vi "Database Configuration.vi"() -> ()   [LabVIEW 2023, in "GUI.lvlib" / "Diagnostic.lvlib"]
uses:
  Diagnostic.lvlib
  HardwareAbstractionLayer_LVOOP/Database/SQL Public VI/Control/DB Options.ctl
  <vilib>/Utility/file.llb/Write Delimited Spreadsheet (string).vi
  <vilib>/Utility/file.llb/Read Delimited Spreadsheet (string).vi
  HardwareAbstractionLayer_LVOOP/Database/Database.lvclass
panel:
  out "PhysicalChannel":string
  in  "Search":bool
  in  "Update":bool
  in  "Tab Control":enum32{"DAQ", "Database"}(tab)
  in  "DAQ":i32(listbox)
  in  "Signal Name":string(combo)
  in  "Enabled":bool
  in  "Channel Type":string(combo)
  in  "DUT ID":string(combo)
  in  "List Table Name":string(combo)
  in  "List Schema":string(combo)
  in  "Selection":string(combo)
  in  "Export":bool
  in  "Import":bool
  in  "Database":i32(listbox)
  in  "Exit":bool
  out "error out":errorcluster
  in  "error in":errorcluster
  # "Database Configuration"
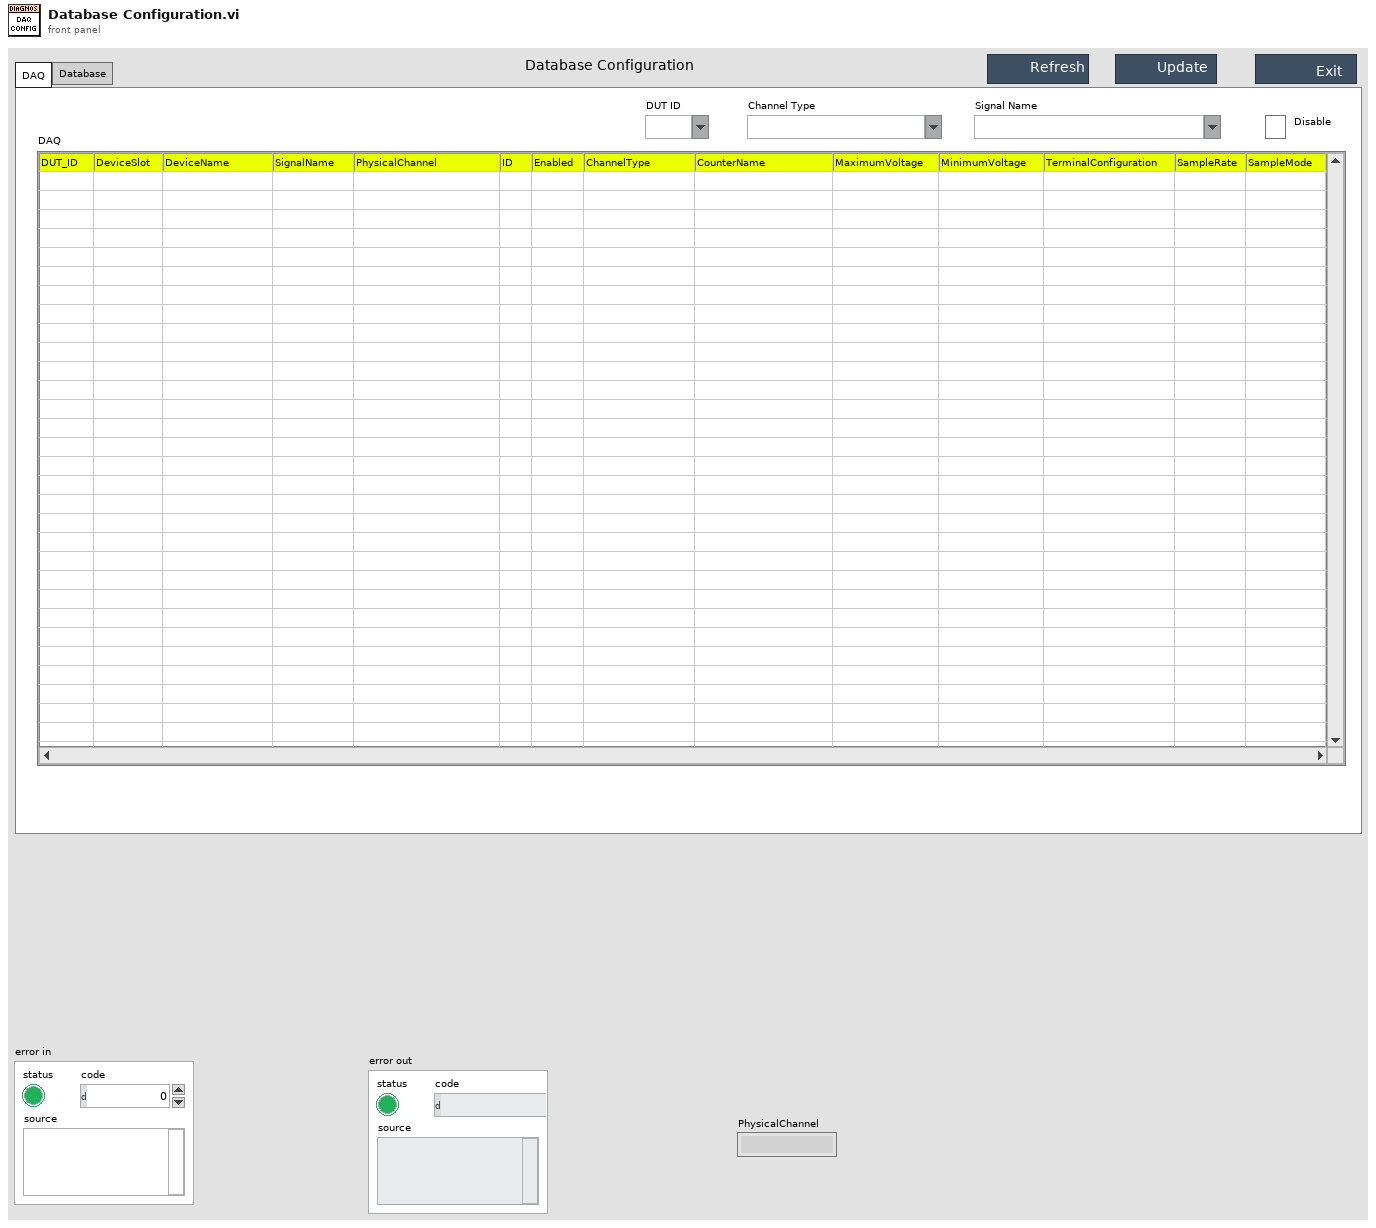
[diagram p1: front panel]
types:
  T1 = typedef "HardwareAbstractionLayer_LVOOP.lvlib/Database.lvclass/DB Options.ctl" = enum16{"Init", "Select Data", "Insert Data", "Update Data", "Delete Data", "Execute Query", "Create Schema", "Create Table", "List Tables", "List Columns", "Close"}
  T2 = cluster{"table":string, "columns":string[], "Data":string[][], "Schema Name":string}
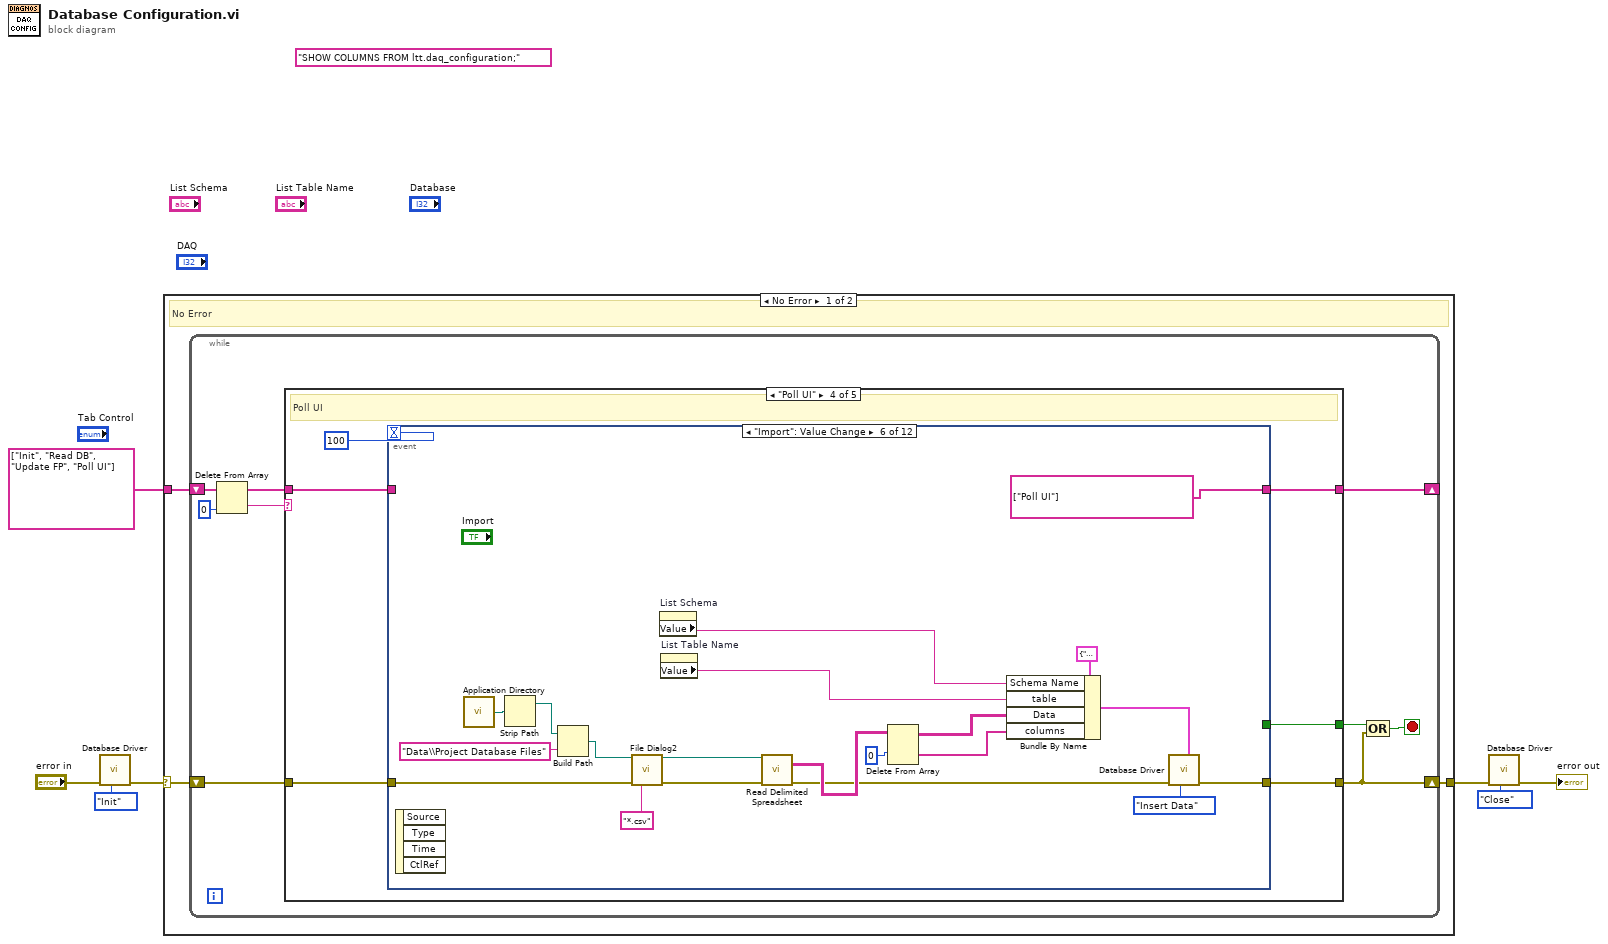
[diagram p0: block diagram]
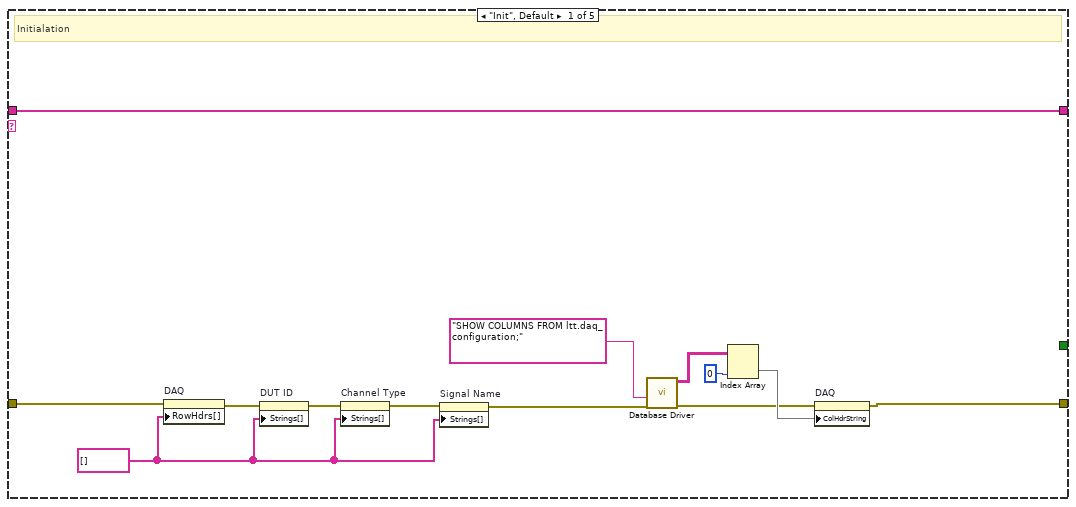
[diagram p2: hidden frame]
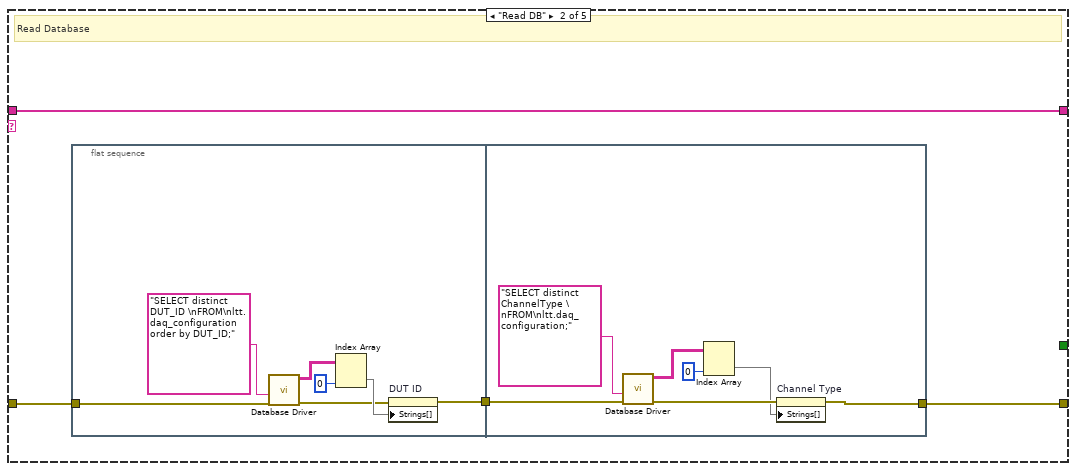
[diagram p3: hidden frame]
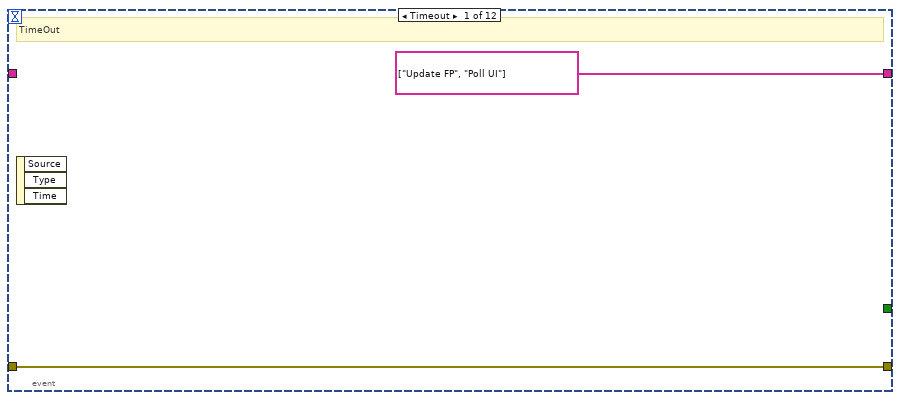
[diagram p5: hidden frame]
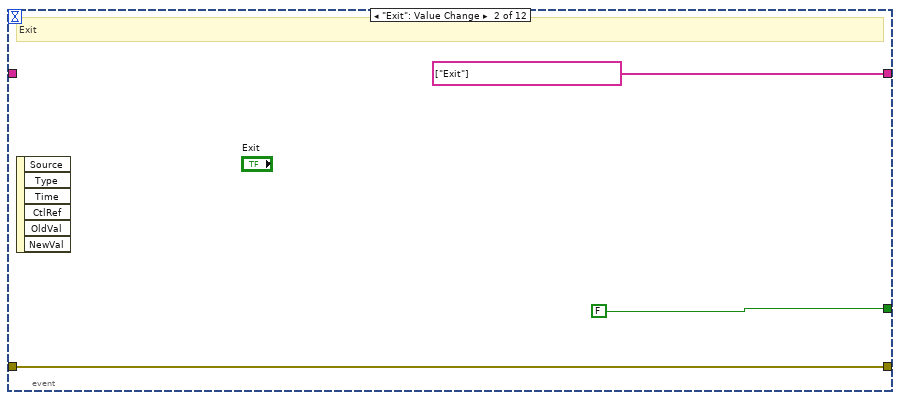
[diagram p6: hidden frame]
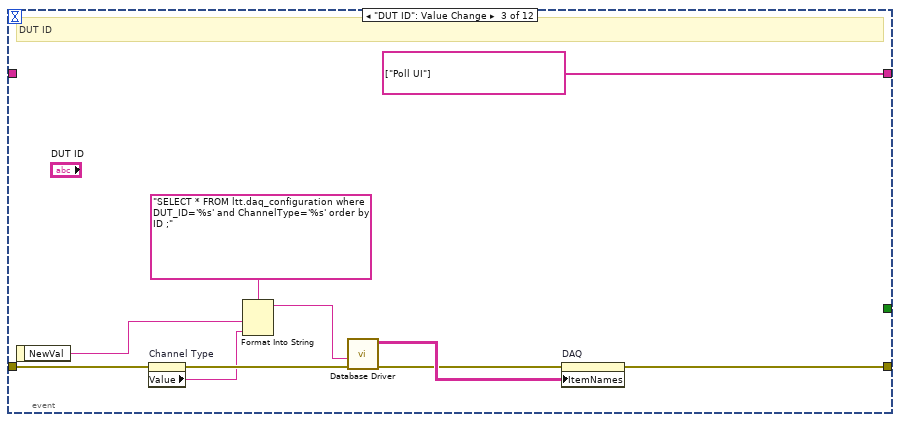
[diagram p7: hidden frame]
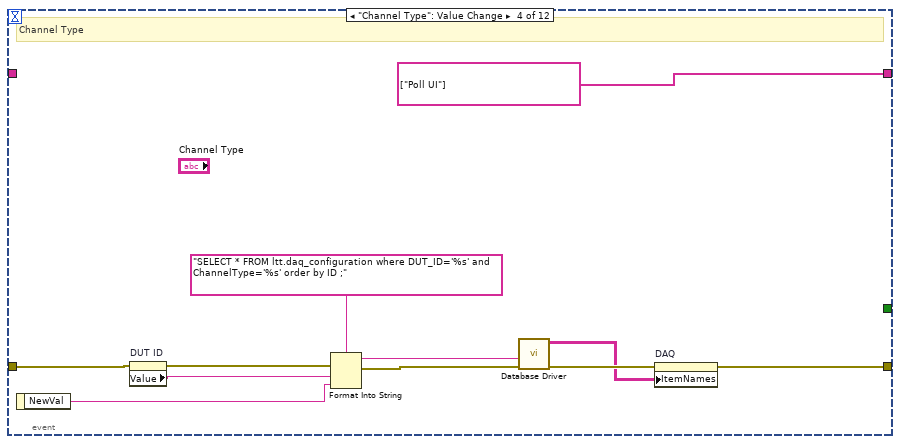
[diagram p8: hidden frame]
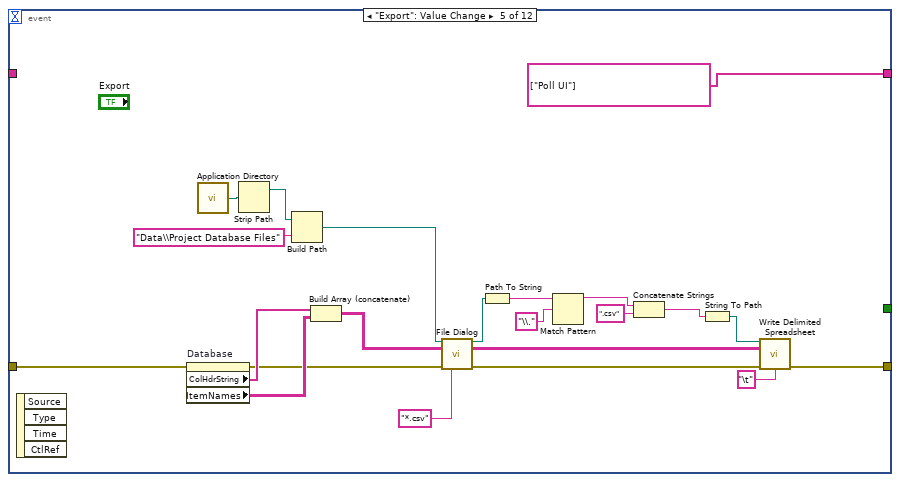
[diagram p9: hidden frame]
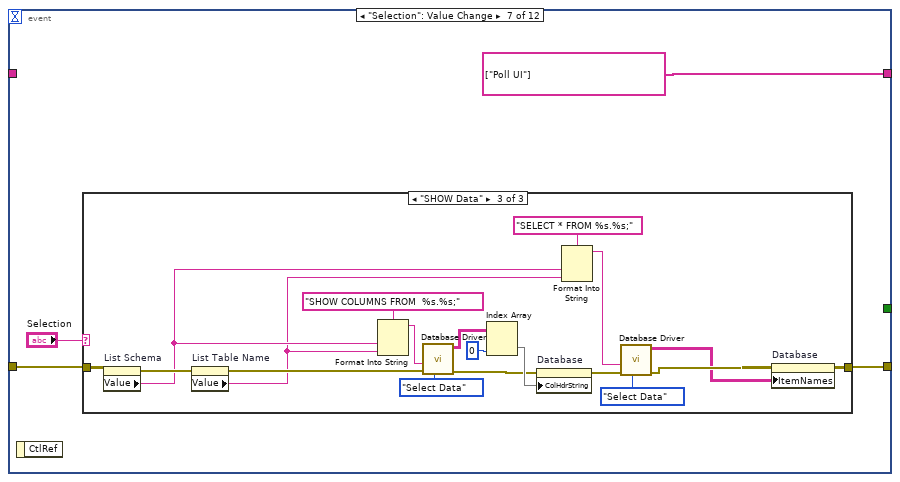
[diagram p10: hidden frame]
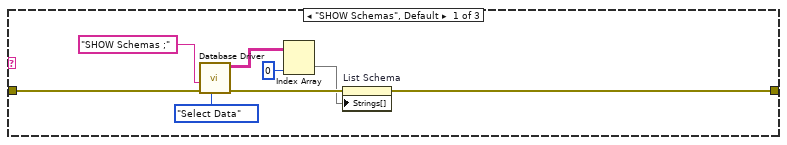
[diagram p11: hidden frame]
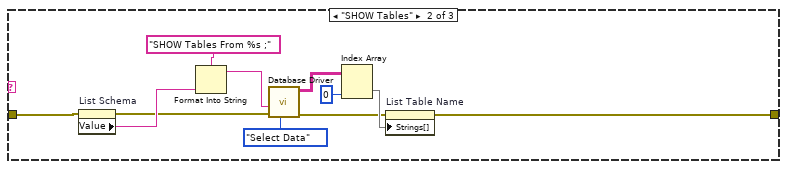
[diagram p12: hidden frame]
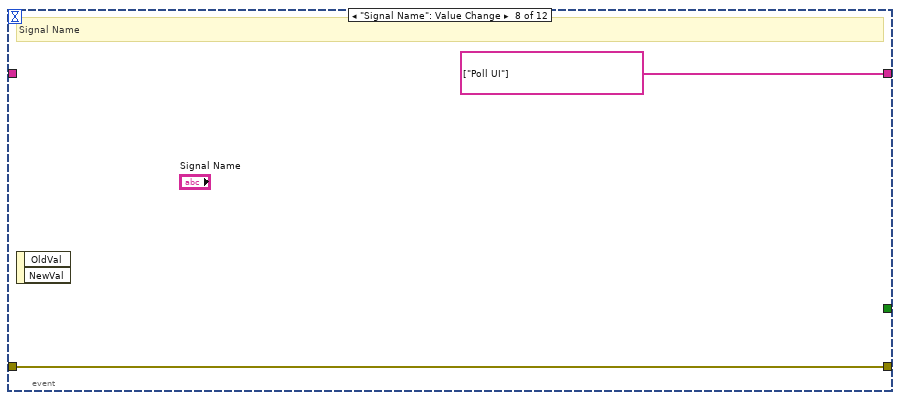
[diagram p13: hidden frame]
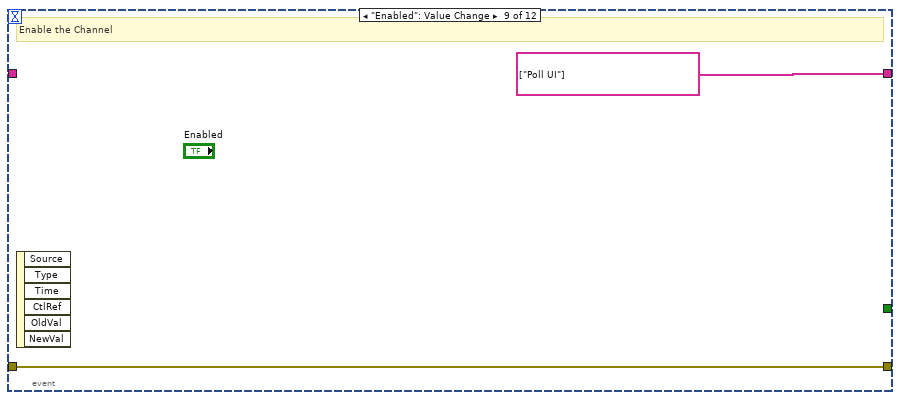
[diagram p14: hidden frame]
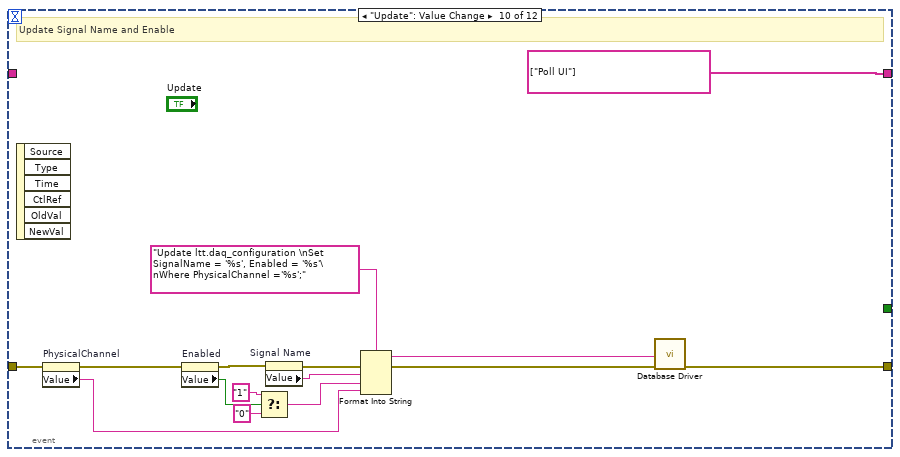
[diagram p15: hidden frame]
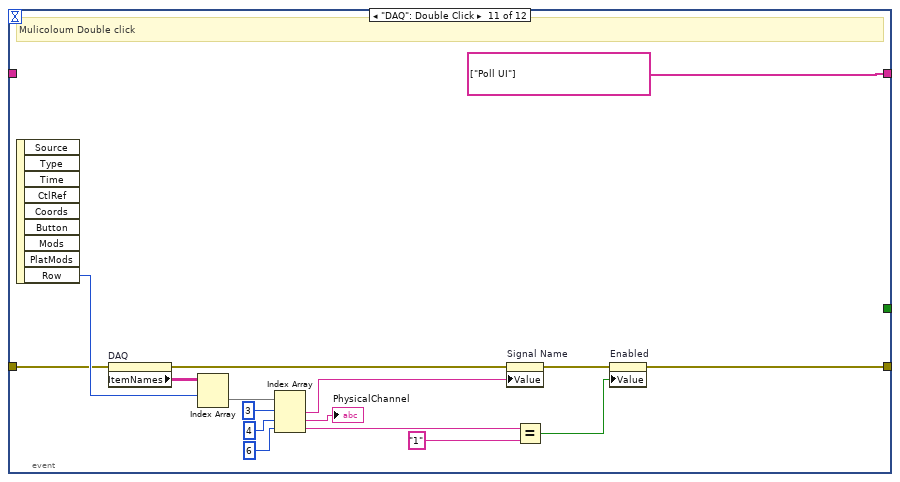
[diagram p16: hidden frame]
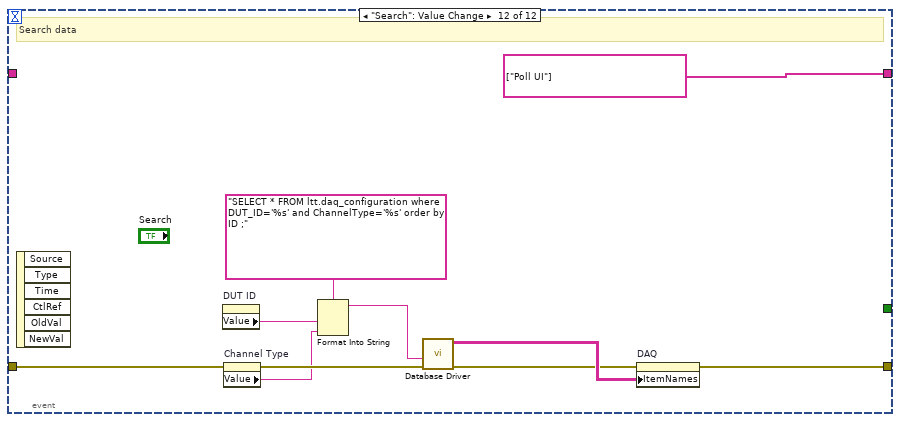
[diagram p17: hidden frame]
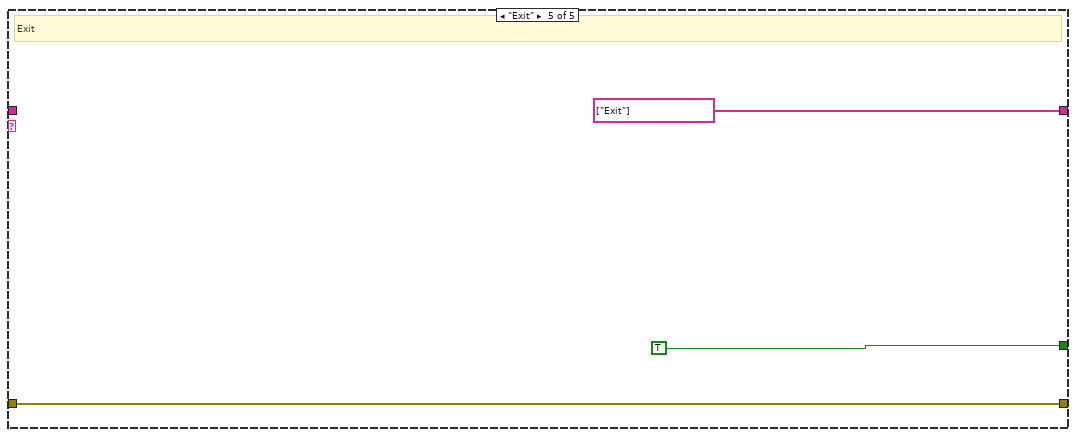
[diagram p18: hidden frame]
diagram:
  (unwired) "SHOW COLUMNS FROM ltt.daq_configuration;" ("SQL query")
  n1 = call "Database Driver.vi"("Options"=DB_Options."Init", "error in"="error in") -> ("error out"=w3:errorcluster)  [unwired: 6 in, 3 out]
  n2 = case shown="No Error" w3 {
    selector: w3 -> [w10 w216]
    tunnel: [w9 w216] -> w2
    tunnel: string[] ["Init", "Read DB", "Update FP", "Poll UI"] -> [w8 _]
    frame No Error {
      # "No Error"
      n3 = while {
        shift-right: [w11] -> w9
        shift-left: w10 -> [w19]
        shift-right: [w15] -> _
        shift-left: w8 -> [w18]
        stop <- w12 stop-if-true
        n4 = Delete From Array(array=w18, index=0) -> (deleted portion=w17:string, array with subset deleted=w16:string[])  [unwired: 1 in]
        n5 = case shown="\"Poll UI\"" w17 {
          tunnel: w19 -> [w31 w35 w51 w58 w214]
          tunnel: [w20 w34 w51 w57 w214] -> w11
          tunnel: w16 -> [w32 w36 w52 w54 _]
          tunnel: [w32 w36 w52 w53 string[] ["Exit"]] -> w15
          tunnel: [_ _ _ w55 TRUE] -> w14
          frame "Init", Default {
            w27 = string[] [] ("Row Header Strings[]")
            # "Initialation"
            n6 = property on="DAQ" class="MCListbox (strict)"(error in=w31, "RowHdrs[]"=w27) -> (error out=w30:errorcluster)  [unwired: 1 in, 1 out]
            n7 = property on="DUT ID" class="CmbBox"(error in=w30, "Strings[]"=w27) -> (error out=w29:errorcluster)  [unwired: 1 in, 1 out]
            n8 = property on="Channel Type" class="CmbBox"(error in=w29, "Strings[]"=w27) -> (error out=w28:errorcluster)  [unwired: 1 in, 1 out]
            n9 = property on="Signal Name" class="CmbBox"(error in=w28, "Strings[]"=w27) -> (error out=w26:errorcluster)  [unwired: 1 in, 1 out]
            n10 = call "Database Driver.vi"("error in"=w26, "SQL query"="SHOW COLUMNS FROM ltt.daq_configuration;") -> ("error out"=w21:errorcluster, "data"=w24:string[][])  [unwired: 6 in, 2 out]
            n11 = Index Array(array=w24, index (col)=0 ("disabled index (col)")) -> (element=w22:string[])  [unwired: 1 in]
            n12 = property on="DAQ" class="MCListbox (strict)"(error in=w21, "ColHdrString"=w22) -> (error out=w20:errorcluster)  [unwired: 1 in, 1 out]
          }
          frame "Read DB" {
            # "Read Database"
            n13 = flat-sequence {
              tunnel: w35 -> [w43]
              tunnel: [w37] -> w33
              tunnel: [w45] -> w34
              tunnel: w33 -> [w47]
              frame #0 {
                n14 = call "Database Driver.vi"("error in"=w43, "SQL query"="SELECT distinct DUT_ID \nFROM\nltt.daq_configuration order by DUT_ID;") -> ("error out"=w38:errorcluster, "data"=w41:string[][])  [unwired: 6 in, 2 out]
                n15 = Index Array(array=w41, index (col)=0 ("disabled index (col)")) -> (element=w39:string[])  [unwired: 1 in]
                n16 = property on="DUT ID" class="CmbBox"(error in=w38, "Strings[]"=w39) -> (error out=w37:errorcluster)  [unwired: 1 in, 1 out]
              }
              frame #1 {
                n17 = call "Database Driver.vi"("error in"=w47, "SQL query"="SELECT distinct ChannelType \nFROM\nltt.daq_configuration;") -> ("error out"=w46:errorcluster, "data"=w49:string[][])  [unwired: 6 in, 2 out]
                n18 = Index Array(array=w49, index (col)=0 ("disabled index (col)")) -> (element=w44:string[])  [unwired: 1 in]
                n19 = property on="Channel Type" class="CmbBox"(error in=w46, "Strings[]"=w44) -> (error out=w45:errorcluster)  [unwired: 1 in, 1 out]
              }
            }
          }
          frame "Update FP" {
            # "Update Frontpanel"
          }
          frame "Poll UI" {
            # "Poll UI"
            n20 = event shown="[5] \"Import\": Value Change" {
              selector: _ -> [_ _ _ _ _ _ _ _ _ _ _ _]
              dyn-events: _ -> [_ _ _ _ _ _ _ _ _ _ _ _]
              timeout: 100 -> [_ _ _ _ _ _ _ _ _ _ _ _]
              tunnel: w58 -> [w60 w62 w66 w79 w101 w118 w129 w169 w171 w175 w196 w204]
              tunnel: [w60 w62 w68 w82 w104 w117 w128 w169 w171 w182 w192 w203] -> w57
              tunnel: [_ FALSE _ _ _ _ _ _ _ _ _ _] -> w55
              tunnel: w54 -> [_ _ _ _ _ _ _ _ _ _ _ _]
              tunnel: [string[] ["Update FP", "Poll UI"] string[] ["Exit"] string[] ["Poll UI"] string[] ["Poll UI"] string[] ["Poll UI"] string[] ["Poll UI"] string[] ["Poll UI"] string[] ["Poll UI"] string[] ["Poll UI"] string[] ["Poll UI"] string[] ["Poll UI"] string[] ["Poll UI"]] -> w53
              event Timeout {
                # "TimeOut"
                n21 = event-data() -> ()  [unwired: 1 in, 3 out]
              }
              event "Exit": Value Change {
                # "Exit"
                n22 = event-data() -> ()  [unwired: 1 in, 6 out]
              }
              event "DUT ID": Value Change {
                # "DUT ID"
                n23 = event-data() -> ("NewVal"=w72:string)  [unwired: 1 in]
                n24 = property on="Channel Type" class="CmbBox"(error in=w66) -> (error out=w65:errorcluster, "Value"=w64:string)  [unwired: 1 in, 1 out]
                n25 = Format Into String(format string="SELECT * FROM ltt.daq_configuration where DUT_ID='%s' and ChannelType='%s' order by ID ;", w72, w64) -> (resulting string=w71:string)  [unwired: 2 in, 1 out]
                n26 = call "Database Driver.vi"("error in"=w65, "SQL query"=w71) -> ("error out"=w69:errorcluster, "data"=w70:string[][])  [unwired: 6 in, 2 out]
                n27 = property on="DAQ" class="MCListbox (strict)"(error in=w69, "ItemNames"=w70) -> (error out=w68:errorcluster)  [unwired: 1 in, 1 out]
              }
              event "Channel Type": Value Change {
                # "Channel Type"
                n28 = event-data() -> ("NewVal"=w75:string)  [unwired: 1 in]
                n29 = property on="DUT ID" class="CmbBox"(error in=w79) -> (error out=w78:errorcluster, "Value"=w76:string)  [unwired: 1 in, 1 out]
                n30 = Format Into String(format string="SELECT * FROM ltt.daq_configuration where DUT_ID='%s' and ChannelType='%s' order by ID ;", error in=w78, w76, w75) -> (resulting string=w80:string, error out=w77:errorcluster)  [unwired: 1 in]
                n31 = call "Database Driver.vi"("error in"=w77, "SQL query"=w80) -> ("error out"=w84:errorcluster, "data"=w83:string[][])  [unwired: 6 in, 2 out]
                n32 = property on="DAQ" class="MCListbox (strict)"(error in=w84, "ItemNames"=w83) -> (error out=w82:errorcluster)  [unwired: 1 in, 1 out]
              }
              event "Export": Value Change {
                n33 = event-data() -> ()  [unwired: 1 in, 4 out]
                n34 = property on="Database" class="MCListbox (strict)"(error in=w101) -> (error out=w98:errorcluster, "ColHdrString"=w102:string[], "ItemNames"=w103:string[][])  [unwired: 1 in, 1 out]
                n35 = call <vilib>:"Application Directory.vi"() -> ("Application Directory"=w96:path)
                n36 = Strip Path(path=w96) -> (stripped path=w95:path)  [unwired: 1 out]
                n37 = Build Path(base path=w95, name or relative path="Data\\Project Database Files") -> (appended path=w93:path)
                n38 = Build Array (concatenate)(w102, w103) -> (w100:string[][])
                n39 = call "File Dialog"("start path"=w93, "error in"=w98, "pattern (all files)"="*.csv") -> ("selected path"=w91:path, "error out"=w97:errorcluster)  [unwired: 9 in, 2 out]
                n40 = Path To String(path=w91) -> (string=w90:string)
                n41 = Match Pattern(string=w90, regular expression="\\." ("pattern (all files)")) -> (before substring=w88:string)  [unwired: 1 in, 3 out]
                n42 = Concatenate Strings(w88, ".csv" ("string")) -> (w86:string)
                n43 = String To Path(string=w86) -> (path=w85:path)
                n44 = call-poly <vilib>:"Write Delimited Spreadsheet.vi"("file path (dialog if empty)"=w85, "2D data"=w100, "error in (no error)"=w97, "delimiter (\\t)"="\t" ("delimiter (\\t)")) -> ("error out"=w104:errorcluster)  [unwired: 10 in, 1 out]
              }
              event "Import": Value Change {
                n45 = event-data() -> ()  [unwired: 1 in, 4 out]
                n46 = call <vilib>:"Application Directory.vi"() -> ("Application Directory"=w113:path)
                n47 = Strip Path(path=w113) -> (stripped path=w112:path)  [unwired: 1 out]
                n48 = Build Path(base path=w112, name or relative path="Data\\Project Database Files") -> (appended path=w110:path)
                n49 = call "File Dialog2"("start path"=w110, "error in"=w118, "pattern (all files)"="*.csv" ("pattern label")) -> ("selected path"=w115:path, "error out"=w116:errorcluster)  [unwired: 9 in, 2 out]
                n50 = property on="List Schema" class="CmbBox"() -> ("Value"=w106:string)  [unwired: 2 in, 2 out]
                n51 = property on="List Table Name" class="CmbBox"() -> ("Value"=w107:string)  [unwired: 2 in, 2 out]
                n52 = call-poly <vilib>:"Read Delimited Spreadsheet.vi"("file path (dialog if empty)"=w115, "error in (no error)"=w116) -> ("all rows"=w123:string[][], "error out"=w119:errorcluster)  [unwired: 8 in, 4 out]
                n53 = Delete From Array(array=w123, index (row)=0) -> (deleted portion=w121:string[], array with subset deleted=w122:string[][])  [unwired: 2 in]
                n54 = Bundle By Name(cluster=T2 {"table"="", "columns"=[], "Data"=[], "Schema Name"=""} ("Insert Data"), "Schema Name"=w106, "table"=w107, "Data"=w122, "columns"=w121) -> (w108:T2)
                n55 = call "Database Driver.vi"("Insert Data"=w108, "Options"=DB_Options."Insert Data", "error in"=w119) -> ("error out"=w117:errorcluster)  [unwired: 5 in, 3 out]
              }
              event "Selection": Value Change {
                n56 = event-data() -> ()  [unwired: 1 in, 1 out]
                n57 = case shown="\"SHOW Data\"" "Selection" {
                  tunnel: w129 -> [w135 w144 w162]
                  tunnel: [w131 w139 w159] -> w128
                  frame "SHOW Schemas", Default {
                    n58 = call "Database Driver.vi"("Options"=DB_Options."Select Data", "error in"=w135, "SQL query"="SHOW Schemas ;") -> ("error out"=w132:errorcluster, "data"=w134:string[][])  [unwired: 5 in, 2 out]
                    n59 = Index Array(array=w134, index (col)=0 ("disabled index (col)")) -> (element=w130:string[])  [unwired: 1 in]
                    n60 = property on="List Schema" class="CmbBox"(error in=w132, "Strings[]"=w130) -> (error out=w131:errorcluster)  [unwired: 1 in, 1 out]
                  }
                  frame "SHOW Tables" {
                    n61 = property on="List Schema" class="CmbBox"(error in=w144) -> (error out=w143:errorcluster, "Value"=w145:string)  [unwired: 1 in, 1 out]
                    n62 = Format Into String(format string="SHOW Tables From %s ;" ("SQL query"), w145) -> (resulting string=w146:string)  [unwired: 2 in, 1 out]
                    n63 = call "Database Driver.vi"("Options"=DB_Options."Select Data", "error in"=w143, "SQL query"=w146) -> ("error out"=w140:errorcluster, "data"=w142:string[][])  [unwired: 5 in, 2 out]
                    n64 = Index Array(array=w142, index (col)=0 ("disabled index (col)")) -> (element=w141:string[])  [unwired: 1 in]
                    n65 = property on="List Table Name" class="CmbBox"(error in=w140, "Strings[]"=w141) -> (error out=w139:errorcluster)  [unwired: 1 in, 1 out]
                  }
                  frame "SHOW Data" {
                    n66 = property on="List Schema" class="CmbBox"(error in=w162) -> (error out=w161:errorcluster, "Value"=w150:string)  [unwired: 1 in, 1 out]
                    n67 = property on="List Table Name" class="CmbBox"(error in=w161) -> (error out=w160:errorcluster, "Value"=w149:string)  [unwired: 1 in, 1 out]
                    n68 = Format Into String(format string="SHOW COLUMNS FROM  %s.%s;" ("SQL query"), w150, w149) -> (resulting string=w167:string)  [unwired: 2 in, 1 out]
                    n69 = call "Database Driver.vi"("Options"=DB_Options."Select Data", "error in"=w160, "SQL query"=w167) -> ("error out"=w157:errorcluster, "data"=w166:string[][])  [unwired: 5 in, 2 out]
                    n70 = Index Array(array=w166, index (col)=0 ("disabled index (col)")) -> (element=w158:string[])  [unwired: 1 in]
                    n71 = property on="Database" class="MCListbox (strict)"(error in=w157, "ColHdrString"=w158) -> (error out=w155:errorcluster)  [unwired: 1 in, 1 out]
                    n72 = Format Into String(format string="SELECT * FROM %s.%s;", w150, w149) -> (resulting string=w152:string)  [unwired: 2 in, 1 out]
                    n73 = call "Database Driver.vi"("Options"=DB_Options."Select Data", "error in"=w155, "SQL query"=w152) -> ("error out"=w154:errorcluster, "data"=w151:string[][])  [unwired: 5 in, 2 out]
                    n74 = property on="Database" class="MCListbox (strict)"(error in=w154, "ItemNames"=w151) -> (error out=w159:errorcluster)  [unwired: 1 in, 1 out]
                  }
                }
              }
              event "Signal Name": Value Change {
                # "Signal Name"
                n75 = event-data() -> ()  [unwired: 1 in, 2 out]
              }
              event "Enabled": Value Change {
                # "Enable the Channel"
                n76 = event-data() -> ()  [unwired: 1 in, 6 out]
              }
              event "Update": Value Change {
                # "Update Signal Name and Enable"
                n77 = event-data() -> ()  [unwired: 1 in, 6 out]
                n78 = property on="PhysicalChannel" class="Str"(error in=w175) -> (error out=w174:errorcluster, "Value"=w173:string)  [unwired: 1 in, 1 out]
                n79 = property on="Enabled" class="Bool (strict)"(error in=w174) -> (error out=w180:errorcluster, "Value"=w179:bool)  [unwired: 1 in, 1 out]
                n80 = Select(t="1", s=w179, f="0") -> (s? t:f=w177:string)
                n81 = property on="Signal Name" class="CmbBox"(error in=w180) -> (error out=w181:errorcluster, "Value"=w184:string)  [unwired: 1 in, 1 out]
                n82 = Format Into String(format string="Update ltt.daq_configuration \nSet SignalName = '%s', Enabled = '%s'\nWhere PhysicalChannel ='%s';", error in=w181, w184, w177, w173) -> (resulting string=w172:string, error out=w183:errorcluster)  [unwired: 1 in]
                n83 = call "Database Driver.vi"("error in"=w183, "SQL query"=w172) -> ("error out"=w182:errorcluster)  [unwired: 6 in, 3 out]
              }
              event "DAQ": Double Click {
                # "Mulicoloum Double click"
                n84 = event-data() -> ("Row"=w201:i32)  [unwired: 1 in, 8 out]
                n85 = property on="DAQ" class="MCListbox (strict)"(error in=w196) -> (error out=w195:errorcluster, "ItemNames"=w200:string[][])  [unwired: 1 in, 1 out]
                n86 = Index Array(array=w200, index (row)=w201) -> (element=w199:string[])  [unwired: 1 in]
                n87 = Index Array(array=w199, index #1=3 ("index"), index #2=4 ("index"), index #3=6 ("index")) -> (element #1=w197:string, element #2=→"PhysicalChannel":string, element #3=w188:string)
                n88 = property on="Signal Name" class="CmbBox"(error in=w195, "Value"=w197) -> (error out=w193:errorcluster)  [unwired: 1 in, 1 out]
                n89 = Equal?(x=w188, y="1") -> (x = y?=w191:bool)
                n90 = property on="Enabled" class="Bool (strict)"(error in=w193, "Value"=w191) -> (error out=w192:errorcluster)  [unwired: 1 in, 1 out]
              }
              event "Search": Value Change {
                # "Search data"
                n91 = event-data() -> ()  [unwired: 1 in, 6 out]
                n92 = property on="DUT ID" class="CmbBox"() -> ("Value"=w211:string)  [unwired: 2 in, 2 out]
                n93 = property on="Channel Type" class="CmbBox"(error in=w204) -> (error out=w207:errorcluster, "Value"=w206:string)  [unwired: 1 in, 1 out]
                n94 = Format Into String(format string="SELECT * FROM ltt.daq_configuration where DUT_ID='%s' and ChannelType='%s' order by ID ;", w211, w206) -> (resulting string=w210:string)  [unwired: 2 in, 1 out]
                n95 = call "Database Driver.vi"("error in"=w207, "SQL query"=w210) -> ("error out"=w208:errorcluster, "data"=w209:string[][])  [unwired: 6 in, 2 out]
                n96 = property on="DAQ" class="MCListbox (strict)"(error in=w208, "ItemNames"=w209) -> (error out=w203:errorcluster)  [unwired: 1 in, 1 out]
              }
            }
          }
          frame "Exit" {
            # "Exit"
          }
        }
        n97 = Compound Arithmetic op=OR(w14, w11) -> (w12:bool)
      }
    }
    frame Error {
      # "Error"
    }
  }
  n98 = call "Database Driver.vi"("Options"=DB_Options."Close", "error in"=w2) -> ("error out"=→"error out":errorcluster)  [unwired: 6 in, 3 out]
